vi "Fan Acceleration Acquisition.vi"(6 "Acceleration Control Index":i32, 8 "error in":errorcluster, 9 "stop":T1, 10 "Stream":refnum<class "Stream.lvclass">, 11 "DAQmx Task In":refnum<k21>) -> (0 "error out":errorcluster, 3 "DAQmx Task Out":refnum<k21>)   [LabVIEW 2020]
uses:
  submodules/nominal-streaming-labview-ffi/lv_src/Stream/Stream.lvclass
  <extravilib>/ChannelInstances/Tag-bool/))Channel.ctl
  <vilib>/DAQmx/read.llb/DAQmx Read (Analog 1D Wfm NChan NSamp).vi
  <extravilib>/ChannelInstances/Tag-bool/Read With Abort.vi
  <vilib>/DAQmx/miscellaneous.llb/DAQmx Fill In Error Info.vi
  <extravilib>/ChannelInstances/Tag-bool/EndpointRead.vi
  submodules/nominal-streaming-labview-ffi/lv_src/Channel/Channel.lvclass
  <extravilib>/ChannelInstances/Tag-bool.lvlib
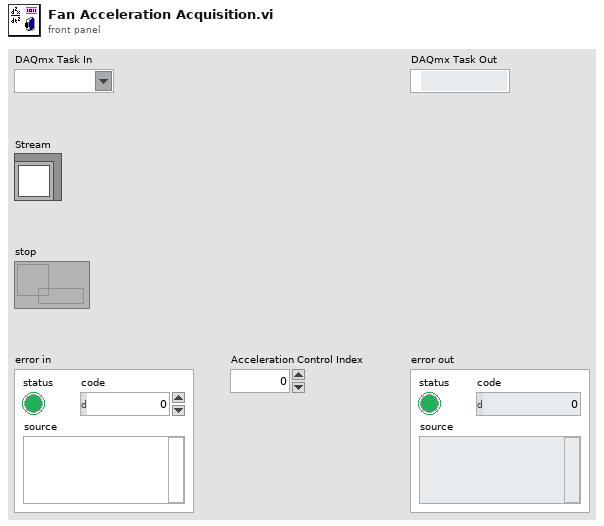
[diagram p1: front panel]
types:
  T1 = typedef "Tag-bool.lvlib/))Channel.ctl" = refnum<queue>
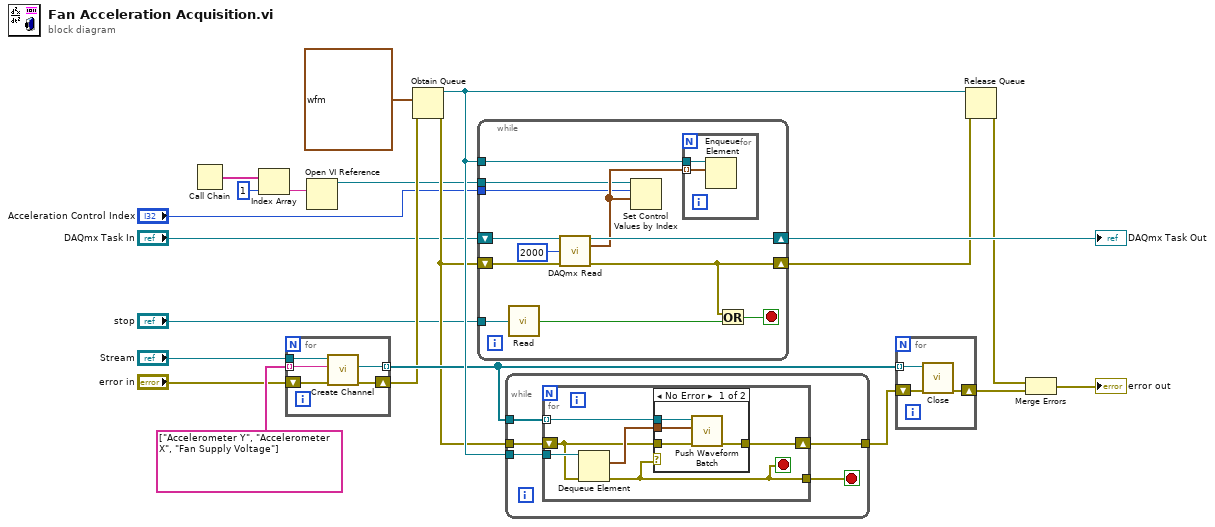
[diagram p0: block diagram]
diagram:
  n1 = Call Chain() -> (call chain=w5:string[])
  n2 = Index Array(array=w5, index=1) -> (element=w3:string)
  n3 = for {
    tunnel: string[] ["Accelerometer Y", "Accelerometer X", "Fan Supply Voltage"] ("Datascope Name") -> [w26] mode=indexing
    tunnel: [w25] -> w17 mode=indexing
    tunnel: "Stream" -> [w24]
    shift-right: [w22] -> w15
    shift-left: "error in" -> [w23]
    n4 = call "Create Channel.vi"("error in (no error)"=w23, "Channel Name"=w26, "Nominal Streaming in"=w24) -> ("error out"=w22:errorcluster, "Channel"=w25:refnum<class "Channel.lvclass">)  [unwired: 6 in, 1 out]
  }
  n5 = Open VI Reference(vi path=w3) -> (vi reference=w2:refnum<vi>)  [unwired: 5 in, 1 out]
  n6 = Obtain Queue(element data type=waveform(dbl) {"t0"=timestamp(0 s since 1904-01-01), "dt"=1.0, "Y"=[]} ("Waveform"), error in (no error)=w15) -> (queue out=w19:refnum<queue>, error out=w14:errorcluster)  [unwired: 3 in, 1 out]
  n7 = while {
    shift-right: [w36] -> w11
    shift-left: "DAQmx Task In" -> [w38]
    shift-right: [w34] -> w8
    shift-left: w14 -> [w37]
    tunnel: w19 -> [w32]
    tunnel: "stop" -> [w31]
    tunnel: w2 -> [w28]
    tunnel: "Acceleration Control Index" -> [w27]
    stop <- w35 stop-if-true
    n8 = call <extravilib>:"Read.vi"("channel"=w31) -> ("element"=w30:bool)  [unwired: 1 in, 1 out]
    n9 = call-poly <vilib>:"DAQmx Read.vi"("task/channels in"=w38, "number of samples per channel"=2000, "error in"=w37) -> ("task out"=w36:refnum<k21>, "data"=w29:waveform(dbl)[], "error out"=w34:errorcluster)  [unwired: 10 in]
    n10 = Set Control Values by Index(0:w28, 1:w27, 2:w29) -> ()  [unwired: 1 in, 1 out]
    n11 = for {
      tunnel: w32 -> [w40]
      tunnel: w29 -> [w39] mode=indexing
      n12 = Enqueue Element(queue=w40, element=w39) -> ()  [unwired: 2 in, 3 out]
    }
    n13 = Or(x=w34, y=w30) -> (x .or. y?=w35:bool)
  }
  "DAQmx Task Out" <- w11
  n14 = while {
    tunnel: w19 -> [w45]
    tunnel: w17 -> [w44]
    tunnel: [w42] -> w16
    tunnel: w14 -> [w43]
    stop <- w41 stop-if-true
    n15 = for {
      tunnel: w45 -> [w51]
      tunnel: w44 -> [w50] mode=indexing
      shift-right: [w48] -> w42
      shift-left: w43 -> [w47]
      tunnel: [w46] -> w41
      stop <- w46 stop-if-true
      n16 = Dequeue Element(queue=w51, error in (no error)=w47) -> (element=w49:waveform(dbl), error out=w46:errorcluster)  [unwired: 1 in, 2 out]
      n17 = case shown="No Error" w46 {
        tunnel: w50 -> [w54 _]
        tunnel: w49 -> [w53 _]
        tunnel: [w55 w56] -> w48
        tunnel: w47 -> [w52 w56]
        frame No Error {
          n18 = call "Push Waveform Batch.vi"("error in (no error)"=w52, "Waveform"=w53, "Channel in"=w54) -> ("error out"=w55:errorcluster)  [unwired: 7 in, 1 out]
        }
        frame Error {
        }
      }
    }
  }
  n19 = for {
    tunnel: w17 -> [w59] mode=indexing
    shift-right: [w57] -> w13
    shift-left: w16 -> [w58]
    n20 = call "Close.vi"("error in (no error)"=w58, "Channel in"=w59) -> ("error out"=w57:errorcluster)  [unwired: 9 in]
  }
  n21 = Release Queue(queue=w19, error in (no error)=w8) -> (error out=w7:errorcluster)  [unwired: 1 in, 2 out]
  n22 = Merge Errors(w7, w13) -> (→"error out":errorcluster)
